vi "ResetSolenoid.vi"(8 "error in (no error)":errorcluster, 11 "DoubleSolenoid in":refnum<class "DoubleSolenoid.lvclass">) -> (0 "error out":errorcluster, 3 "DoubleSolenoid out":refnum<class "DoubleSolenoid.lvclass">)   [LabVIEW 2018, in "Pneumatics control.lvlib" / "DoubleSolenoid.lvclass"]
doc: "This VI moves all of our pneumatic to the reverse state so its known what state they are in. This code is blocking for 50 ms*"
uses:
  DoubleSolenoid.lvclass
  C:/Users/Howdy Bots/Documents/2019DeepSpace/Classes/Pnematics control/Solenoids/Solenoids.lvclass
  <vilib>/Rock Robotics/WPI/Solenoid/WPI_SolenoidValue.ctl
  DoubleSolenoid.lvclass/DoubleSolenoid.ctl
  <vilib>/Rock Robotics/WPI/Solenoid/WPI_SolenoidSetEnum.vi
  Solenoids.lvclass
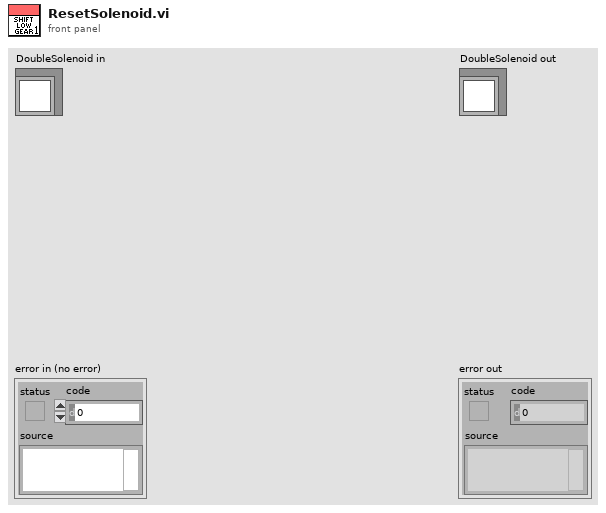
[diagram p1: front panel]
types:
  T1 = typedef "WPI_SolenoidValue.ctl" = enum16{"Off", "On", "Forward", "Reverse"}
  T2 = typedef "WPI_SolenoidDevRef.ctl" = cluster{"DevStatus":errorcluster, "Pneumatics Control Module":u8, "Forward Solenoid Channel":T3, "Reverse Solenoid Channel":T3}
  T3 = typedef "WPI_SolenoidChannel.ctl" = enum8{"Solenoid 0", "Solenoid 1", "Solenoid 2", "Solenoid 3", "Solenoid 4", "Solenoid 5", "Solenoid 6", "Solenoid 7", "Invalid"}
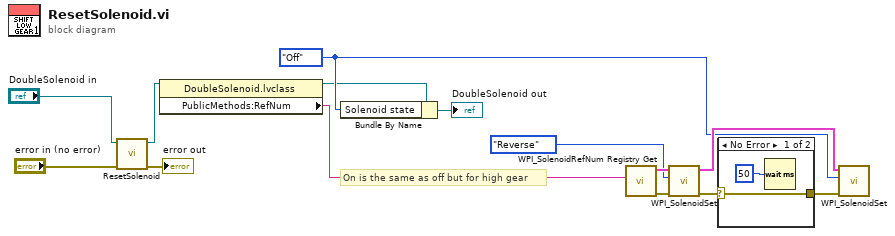
[diagram p0: block diagram]
diagram:
  w4 = WPI_SolenoidValue."Off" ("Value")
  # "On is the same as off but for high gear"
  n1 = call-parent "ResetSolenoid.vi"("error in (no error)"="error in (no error)", "Solenoids in"="DoubleSolenoid in") -> ("error out"=→"error out":errorcluster, "Solenoids out"=w10:refnum<class "DoubleSolenoid.lvclass">)  [unwired: 8 in]
  n2 = property class="DoubleSolenoid.lvclass"(reference=w10) -> (reference out=w2:refnum<class "DoubleSolenoid.lvclass">, "PublicMethods:RefNum"=w11:string)  [unwired: 1 in, 1 out]
  n3 = Bundle By Name(cluster=w2, "Solenoid state"=w4) -> (→"DoubleSolenoid out":refnum<class "DoubleSolenoid.lvclass">)
  n4 = call <vilib>:"WPI_SolenoidRefNum Registry Get.vi"("refnum name"=w11) -> ("error out"=w8:errorcluster, "SolenoidDevRef"=w9:T2)  [unwired: 9 in]
  n5 = call-poly <vilib>:"WPI_SolenoidSet.vi"("error in (no error)"=w8, "Value"=WPI_SolenoidValue."Reverse", "SolenoidDevRef"=w9) -> ("error out"=w6:errorcluster, "SolenoidDevRef"=w5:T2)  [unwired: 7 in]
  n6 = case shown="No Error" w6 {
    selector: w6 -> [w15 w17]
    tunnel: [w15 w17] -> w3
    frame No Error {
      n7 = Wait (ms)(milliseconds to wait=u32 50) -> ()  [unwired: 1 out]
    }
    frame Error {
    }
  }
  n8 = call-poly <vilib>:"WPI_SolenoidSet.vi"("error in (no error)"=w3, "Value"=w4, "SolenoidDevRef"=w5) -> ()  [unwired: 7 in, 2 out]
